vi "Building Array for 3.0.vi"(0 "Number of y":dbl, 1 "Number of x":dbl, 2 "Timepoints":dbl[](array[numeric]), 3 "Folder to Save":path, 4 "No. of Gr":i32, 5 "No. of Sets":i32, 6 "Name of File":string, 7 "Folder Name":string) -> ()   [LabVIEW 2015]
uses:
  <vilib>/Utility/file.llb/Read Delimited Spreadsheet (DBL).vi
  <vilib>/Utility/file.llb/Write Delimited Spreadsheet (DBL).vi
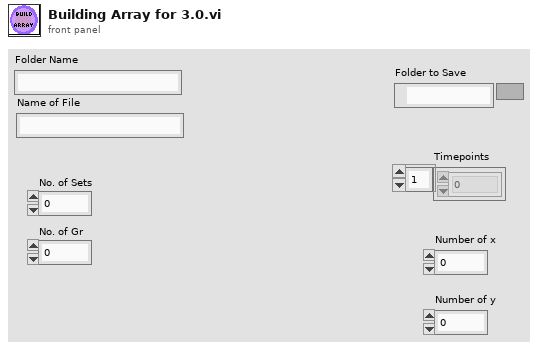
[diagram p1: front panel]
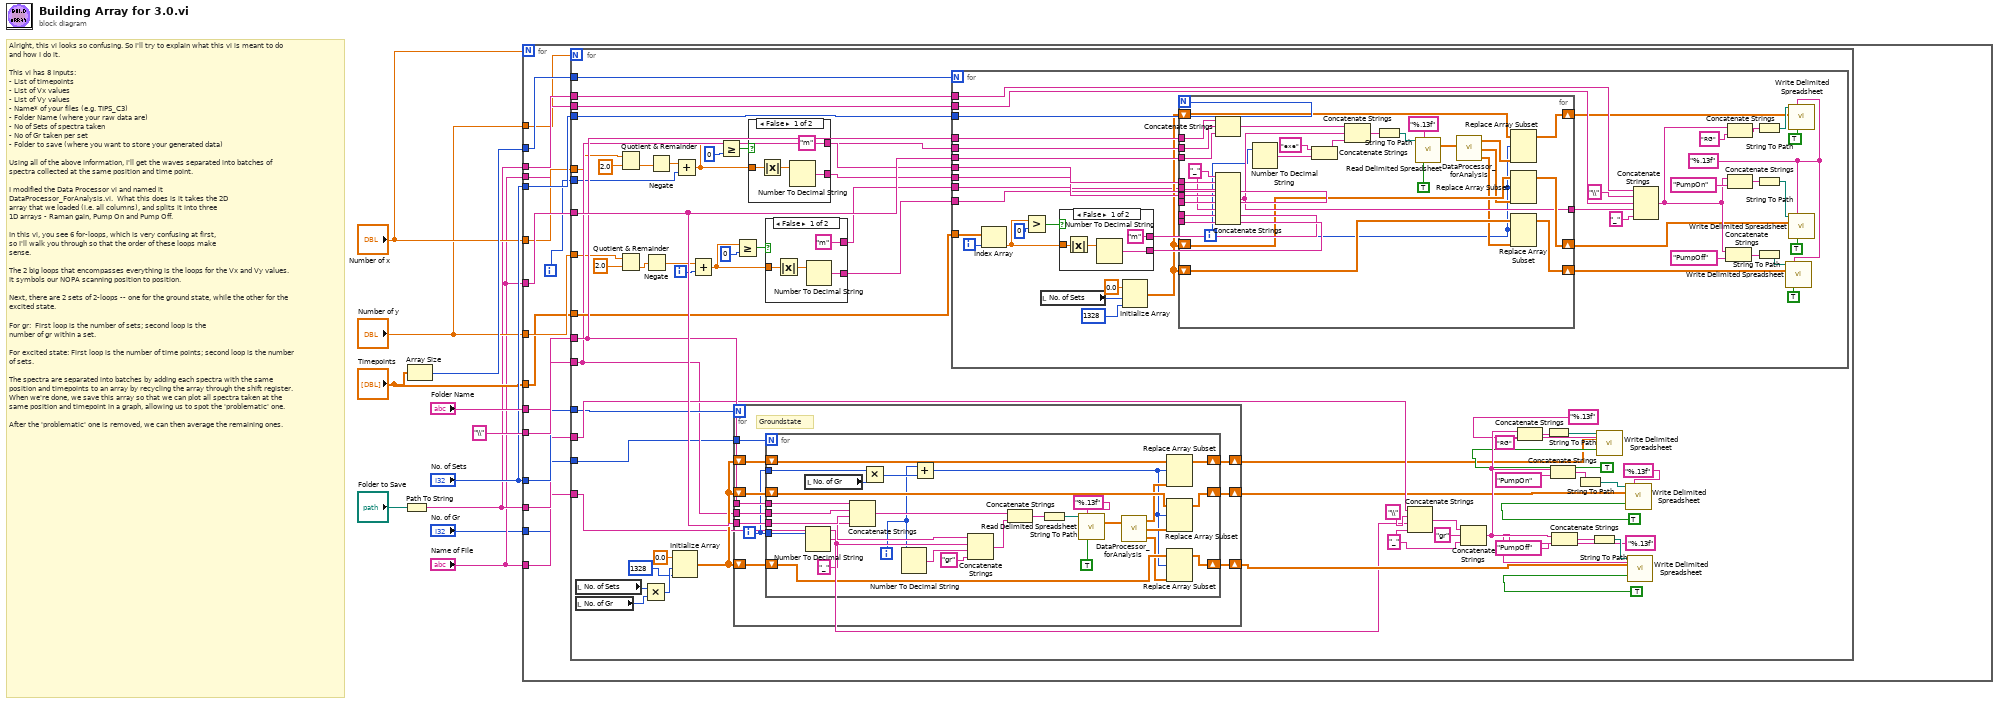
[diagram p0: block diagram]
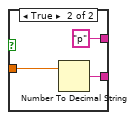
[diagram p2: hidden frame]
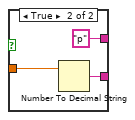
[diagram p3: hidden frame]
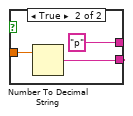
[diagram p4: hidden frame]
diagram:
  # "Alright, this vi looks so confusing. So I'll try to explain what this vi is meant to do and how I do it.\n\nThis vi has 8 inputs:\n- List of timepoints \n- List of Vx values \n- List of Vy values\n- Name* of your files (e.g. TIPS_C3)\n- Folder Name (where your raw data are)\n- No of Sets of spectra taken\n- No of Gr taken per set\n- Folder to save (where you want to store your generated data)\n\nUsing all of the above information, I'll get the waves separated into batches of spectra collected at the same position and time point.\n\nI modified the Data Processor vi and named it\nDataProcessor_ForAnalysis.vi.  What this does is it takes the 2D\narray that we loaded (i.e. all columns), and splits it into three\n1D arrays - Raman gain, Pump On and Pump Off.\n\nIn this vi, you see 6 for-loops, which is very confusing at first,\nso I'll walk you through so that the order of these loops make \nsense. \n\nThe 2 big loops that encompasses everything is the loops for the Vx and Vy values.  It symbols our NOPA scanning position to position.\n\nNext, there are 2 sets of 2-loops -- one for the ground state, while the other for the excited state.\n\nFor gr:  First loop is the number of sets; second loop is the\nnumber of gr within a set.\n\nFor excited state: First loop is the number of time points; second loop is the number of sets.\n\nThe spectra are separated into batches by adding each spectra with the same position and timepoints to an array by recycling the array through the shift register. When we're done, we save this array so that we can plot all spectra taken at the same position and timepoint in a graph, allowing us to spot the 'problematic' one. \n\nAfter the 'problematic' one is removed, we can then average the remaining ones."
  n1 = Path To String(path="Folder to Save") -> (string=w3:string)
  n2 = Array Size(array="Timepoints") -> (size(s)=w9:i32)
  n3 = for {
    N: "Number of x" -> [_]
    tunnel: "Name of File" -> [w27]
    tunnel: "\\" -> [w26]
    tunnel: "Folder Name" -> [w25]
    tunnel: "Number of y" -> [w13]
    tunnel: w9 -> [w24]
    tunnel: "No. of Sets" -> [w23]
    tunnel: "No. of Sets" -> [w22]
    tunnel: "Number of x" -> [w21]
    tunnel: "Number of y" -> [w19]
    tunnel: "Timepoints" -> [w18]
    tunnel: w3 -> [w17]
    tunnel: w3 -> [w16]
    tunnel: "Name of File" -> [w15]
    tunnel: "Name of File" -> [w14]
    tunnel: "No. of Gr" -> [w12]
    i -> [w20]
    n4 = for {
      N: w13 -> [_]
      tunnel: w27 -> [w88]
      tunnel: w26 -> [w44]
      tunnel: w25 -> [w87]
      tunnel: w24 -> [w86]
      tunnel: w23 -> [w85]
      tunnel: w22 -> [w46]
      tunnel: w21 -> [w36]
      tunnel: w20 -> [w35]
      tunnel: w19 -> [w28]
      tunnel: w18 -> [w74]
      tunnel: w17 -> [w73]
      tunnel: w16 -> [w72]
      tunnel: w15 -> [w40]
      tunnel: w14 -> [w56]
      tunnel: w12 -> [w43]
      i -> [w79]
      w52 = "_" ("string")
      n5 = local read "No. of Sets"() -> (w42:i32)
      n6 = local read "No. of Gr"() -> (w41:i32)
      n7 = Quotient & Remainder(x=w36, y=2.0) -> (floor(x/y)=w29:dbl)  [unwired: 1 out]
      n8 = Quotient & Remainder(x=w28, y=2.0) -> (floor(x/y)=w32:dbl)  [unwired: 1 out]
      n9 = Multiply(x=w42, y=w41) -> (x*y=w39:i32)
      n10 = Negate(x=w32) -> (-x=w31:dbl)
      n11 = Negate(x=w29) -> (-x=w34:dbl)
      n12 = Initialize Array(0.0 ("element"), w39, 1328 ("dimension size")) -> (w45:dbl[][])
      n13 = Add(x=w34, y=w35) -> (x+y=w37:dbl)
      n14 = Add(x=w31, y=w79) -> (x+y=w80:dbl)
      n15 = Greater Or Equal?(x=w37, y=0) -> (x >= y?=w83:bool)
      n16 = for {
        N: w46 -> [_]
        tunnel: w88 -> [w113]
        tunnel: w44 -> [w112]
        tunnel: w87 -> [w111]
        tunnel: w43 -> [w110]
        shift-right: [w109] -> w48
        shift-left: w45 -> [w106]
        shift-right: [w108] -> w50
        shift-left: w45 -> [w105]
        shift-right: [w107] -> w49
        shift-left: w45 -> [w104]
        i -> [w103]
        # "Groundstate"
        n17 = for {
          N: w110 -> [_]
          tunnel: w113 -> [w139]
          tunnel: w112 -> [w140]
          tunnel: w111 -> [w141]
          tunnel: w103 -> [w142]
          shift-right: [w123] -> w109
          shift-left: w106 -> [w122]
          shift-right: [w124] -> w107
          shift-left: w104 -> [w125]
          shift-right: [w127] -> w108
          shift-left: w105 -> [w126]
          tunnel: w103 -> [w120]
          i -> [w114]
          w137 = "_"
          n18 = local read "No. of Gr"() -> (w121:i32)
          n19 = Number To Decimal String(number=w142) -> (decimal integer string=w138:string)  [unwired: 1 in]
          n20 = Concatenate Strings(w141, w140, w139, w137) -> (w135:string)
          n21 = Multiply(x=w120, y=w121) -> (x*y=w119:i32)
          n22 = Number To Decimal String(number=w114) -> (decimal integer string=w136:string)  [unwired: 1 in]
          n23 = Add(x=w114, y=w119) -> (x+y=w115:i32)
          n24 = Concatenate Strings(w138, w137, w136, "gr" ("string")) -> (w128:string)
          n25 = Concatenate Strings(w135, w128) -> (w134:string)
          n26 = String To Path(string=w134) -> (path=w131:path)
          n27 = call-poly <vilib>:"Read Delimited Spreadsheet.vi"("file path (dialog if empty)"=w131, "format (%.3f)"="%.13f", "transpose? (F)"=TRUE) -> ("all rows"=w133:dbl[][])  [unwired: 7 in, 5 out]
          n28 = call "DataProcessor_forAnalysis.vi"("Data"=w133) -> ("PumpOff"=w117:dbl[], "PumpOn"=w118:dbl[], "Raman"=w116:dbl[])  [unwired: 3 in]
          n29 = Replace Array Subset(array=w122, new element=w116, index (row)=w115) -> (w123:dbl[][])  [unwired: 1 in]
          n30 = Replace Array Subset(array=w126, new element=w118, index (row)=w115) -> (w127:dbl[][])  [unwired: 1 in]
          n31 = Replace Array Subset(array=w125, new element=w117, index (row)=w115) -> (w124:dbl[][])  [unwired: 1 in]
        }
      }
      n32 = Greater Or Equal?(x=w80, y=0) -> (x >= y?=w82:bool)
      n33 = case shown="False" w83 {
        tunnel: ["m" "p"] -> w78
        tunnel: w37 -> [w99 w100]
        tunnel: [w97 w101] -> w77
        frame False {
          n34 = Absolute Value(x=w99) -> (abs(x)=w98:dbl)
          n35 = Number To Decimal String(number=w98) -> (decimal integer string=w97:string)  [unwired: 1 in]
        }
        frame True {
          n36 = Number To Decimal String(number=w100) -> (decimal integer string=w101:string)  [unwired: 1 in]
        }
      }
      n37 = case shown="False" w82 {
        tunnel: ["m" "p"] -> w76
        tunnel: w80 -> [w91 w93]
        tunnel: [w89 w94] -> w75
        frame False {
          n38 = Absolute Value(x=w91) -> (abs(x)=w90:dbl)
          n39 = Number To Decimal String(number=w90) -> (decimal integer string=w89:string)  [unwired: 1 in]
        }
        frame True {
          n40 = Number To Decimal String(number=w93) -> (decimal integer string=w94:string)  [unwired: 1 in]
        }
      }
      n41 = for {
        N: w86 -> [_]
        tunnel: w88 -> [w183]
        tunnel: w44 -> [w182]
        tunnel: w87 -> [w181]
        tunnel: w85 -> [w170]
        tunnel: w78 -> [w180]
        tunnel: w77 -> [w145]
        tunnel: w76 -> [w179]
        tunnel: w75 -> [w178]
        tunnel: w74 -> [w174]
        tunnel: w73 -> [w162]
        tunnel: w56 -> [w154]
        i -> [w173]
        w151 = "%.13f" ("format (%.3f)")
        n42 = Index Array(array=w174, index=w173) -> (element=w176:dbl)
        n43 = Greater?(x=w176, y=0) -> (0:w175:bool)
        n44 = local read "No. of Sets"() -> (w144:i32)
        n45 = case shown="False" w175 {
          tunnel: ["m" "p"] -> w171
          tunnel: w176 -> [w186 w188]
          tunnel: [w184 w189] -> w172
          frame False {
            n46 = Absolute Value(x=w186) -> (abs(x)=w185:dbl)
            n47 = Number To Decimal String(number=w185) -> (decimal integer string=w184:string)  [unwired: 1 in]
          }
          frame True {
            n48 = Number To Decimal String(number=w188) -> (decimal integer string=w189:string)  [unwired: 1 in]
          }
        }
        n49 = Initialize Array(0.0 ("element"), w144, 1328 ("dimension size")) -> (w146:dbl[][])
        n50 = for {
          N: w170 -> [_]
          tunnel: w183 -> [w211]
          tunnel: w182 -> [w202]
          tunnel: w181 -> [w201]
          tunnel: w180 -> [w217]
          tunnel: w145 -> [w216]
          tunnel: w179 -> [w215]
          tunnel: w178 -> [w214]
          tunnel: w172 -> [w213]
          tunnel: w171 -> [w204]
          shift-right: [w196] -> w148
          shift-left: w146 -> [w195]
          shift-right: [w198] -> w150
          shift-left: w146 -> [w199]
          shift-right: [w212] -> w149
          shift-left: w146 -> [w197]
          tunnel: [w205] -> w156
          i -> [w191]
          w203 = "_"
          n51 = Concatenate Strings(w201, w202, w211) -> (w210:string)
          n52 = Concatenate Strings(w203, w217, w216, w215, w214, w203, w204, w213) -> (w205:string)
          n53 = Number To Decimal String(number=w191) -> (decimal integer string=w208:string)  [unwired: 1 in]
          n54 = Concatenate Strings("exe", w208) -> (w207:string)
          n55 = Concatenate Strings(w210, w205, w207) -> (w206:string)
          n56 = String To Path(string=w206) -> (path=w218:path)
          n57 = call-poly <vilib>:"Read Delimited Spreadsheet.vi"("file path (dialog if empty)"=w218, "format (%.3f)"="%.13f", "transpose? (F)"=TRUE) -> ("all rows"=w220:dbl[][])  [unwired: 7 in, 5 out]
          n58 = call "DataProcessor_forAnalysis.vi"("Data"=w220) -> ("PumpOff"=w192:dbl[], "PumpOn"=w194:dbl[], "Raman"=w193:dbl[])  [unwired: 3 in]
          n59 = Replace Array Subset(array=w199, new element=w193, index (row)=w191) -> (w198:dbl[][])  [unwired: 1 in]
          n60 = Replace Array Subset(array=w197, new element=w194, index (row)=w191) -> (w212:dbl[][])  [unwired: 1 in]
          n61 = Replace Array Subset(array=w195, new element=w192, index (row)=w191) -> (w196:dbl[][])  [unwired: 1 in]
        }
        n62 = Concatenate Strings(w162, "\\" ("string"), w154, w156, "_" ("string")) -> (w152:string)
        n63 = Concatenate Strings(w152, "PumpOff") -> (w153:string)
        n64 = Concatenate Strings(w152, "RG") -> (w165:string)
        n65 = Concatenate Strings(w152, "PumpOn") -> (w163:string)
        n66 = String To Path(string=w165) -> (path=w164:path)
        n67 = String To Path(string=w163) -> (path=w160:path)
        n68 = String To Path(string=w153) -> (path=w159:path)
        n69 = call-poly <vilib>:"Write Delimited Spreadsheet.vi"("file path (dialog if empty)"=w159, "format (%.3f)"=w151, "2D data"=w148, "transpose? (F)"=TRUE) -> ()  [unwired: 10 in, 2 out]
        n70 = call-poly <vilib>:"Write Delimited Spreadsheet.vi"("file path (dialog if empty)"=w164, "format (%.3f)"=w151, "2D data"=w150, "transpose? (F)"=TRUE) -> ()  [unwired: 10 in, 2 out]
        n71 = call-poly <vilib>:"Write Delimited Spreadsheet.vi"("file path (dialog if empty)"=w160, "format (%.3f)"=w151, "2D data"=w149, "transpose? (F)"=TRUE) -> ()  [unwired: 10 in, 2 out]
      }
      n72 = Concatenate Strings(w72, "\\" ("string"), w40, w52) -> (w70:string)
      n73 = Concatenate Strings(w70, "gr" ("string"), w52) -> (w69:string)
      n74 = Concatenate Strings(w69, "RG") -> (w65:string)
      n75 = String To Path(string=w65) -> (path=w61:path)
      n76 = Concatenate Strings(w69, "PumpOn") -> (w64:string)
      n77 = Concatenate Strings(w69, "PumpOff") -> (w63:string)
      n78 = String To Path(string=w64) -> (path=w59:path)
      n79 = String To Path(string=w63) -> (path=w57:path)
      n80 = call-poly <vilib>:"Write Delimited Spreadsheet.vi"("file path (dialog if empty)"=w61, "format (%.3f)"="%.13f", "2D data"=w48, "transpose? (F)"=TRUE) -> ()  [unwired: 10 in, 2 out]
      n81 = call-poly <vilib>:"Write Delimited Spreadsheet.vi"("file path (dialog if empty)"=w59, "format (%.3f)"="%.13f", "2D data"=w50, "transpose? (F)"=TRUE) -> ()  [unwired: 10 in, 2 out]
      n82 = call-poly <vilib>:"Write Delimited Spreadsheet.vi"("file path (dialog if empty)"=w57, "format (%.3f)"="%.13f", "2D data"=w49, "transpose? (F)"=TRUE) -> ()  [unwired: 10 in, 2 out]
    }
  }
